vi "COD质控流程 (子VI).vi"(10 "CODMn量程切换":enum32{"H", "L", "AUTO"}(ring)=enum."AUTO", 11 "COD":bool) -> (2 "CODMn中断报警":bool, 3 "布尔":bool)   [LabVIEW 2016, in "质控单元.lvlib"]
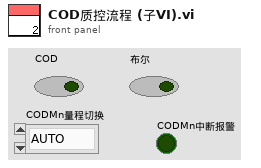
[diagram p1: front panel]
types:
  T1 = enum16{"待机", "启动水样测量", "水样测量中", "启动加标", "启动加标回收", "加标回收测量中", "结束"}
  T2 = cluster{"测量模式":enum16{"水样测量", "标样核查", "零点核查", "跨度核查", "空白测试", "加标回收", "平行样", "校零", "校标"}}
  T3 = cluster{"量程":dbl, "检出限":dbl, "加标前水样浓度":dbl, "加标后水样浓度":dbl, "加标水杯定容体积":dbl, "加标母液浓度":dbl, "加标体积":dbl, "加标回收率":dbl}
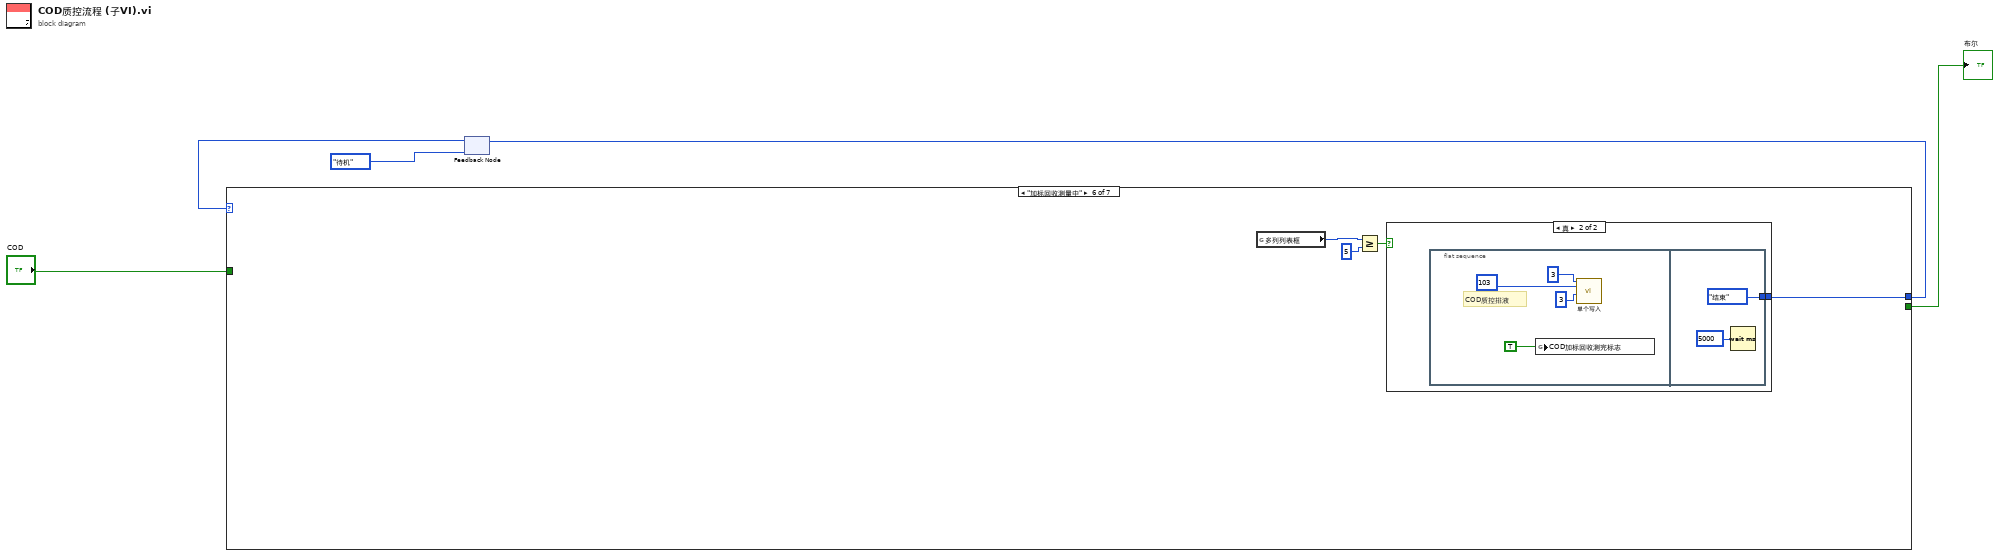
[diagram p0: block diagram]
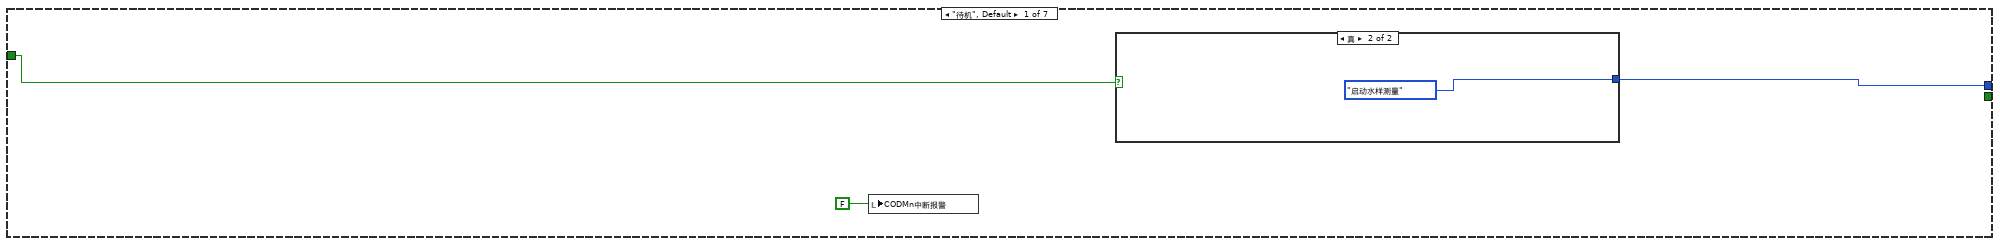
[diagram p2: hidden frame]
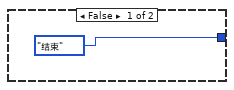
[diagram p3: hidden frame]
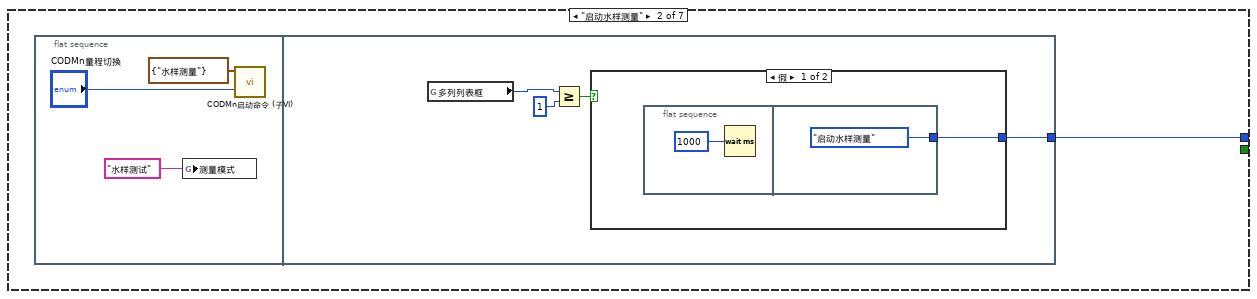
[diagram p4: hidden frame]
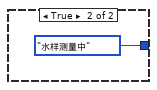
[diagram p5: hidden frame]
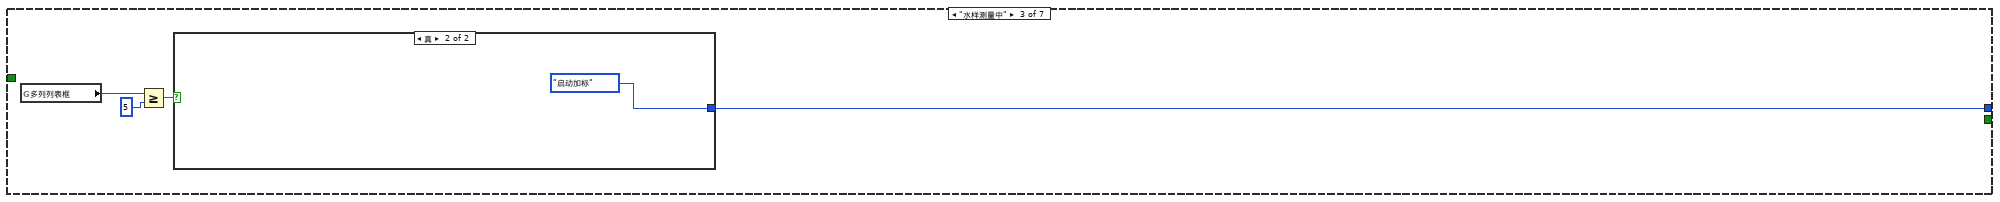
[diagram p6: hidden frame]
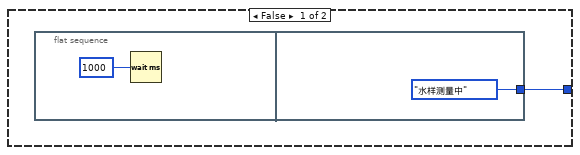
[diagram p7: hidden frame]
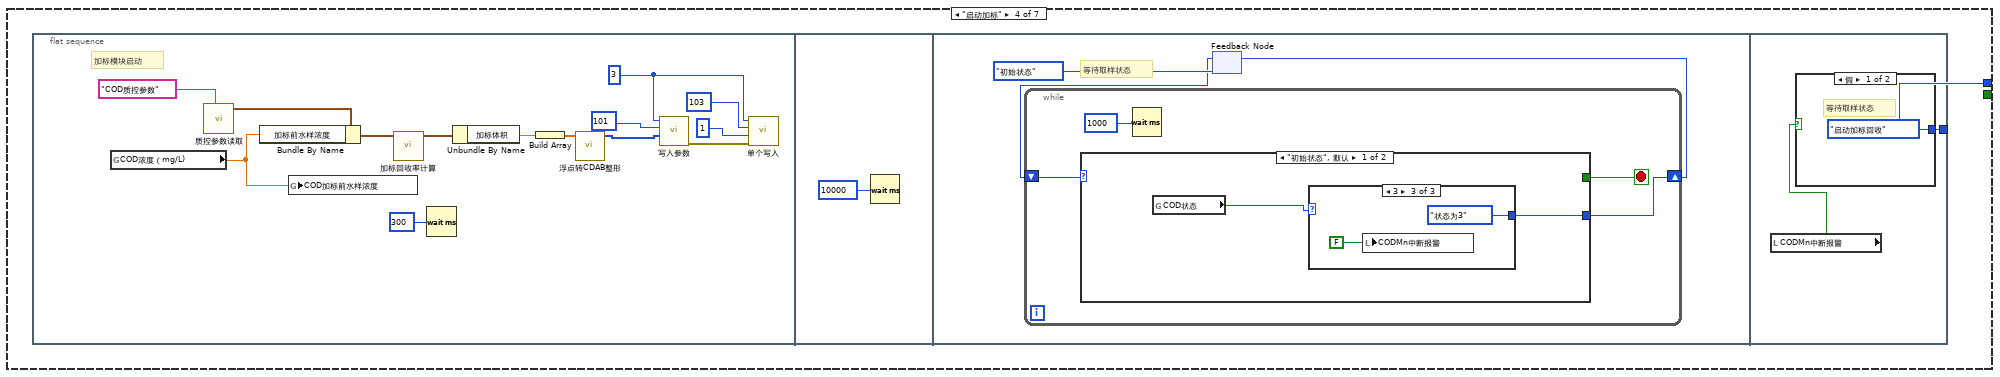
[diagram p8: hidden frame]
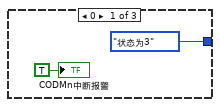
[diagram p9: hidden frame]
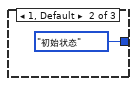
[diagram p10: hidden frame]
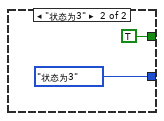
[diagram p11: hidden frame]
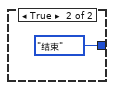
[diagram p12: hidden frame]
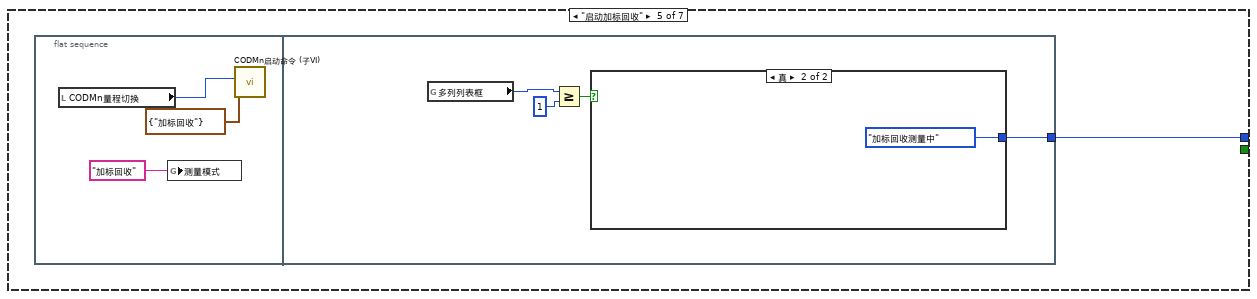
[diagram p13: hidden frame]
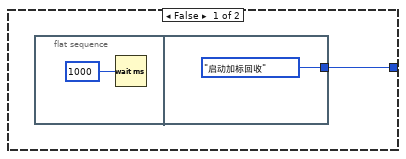
[diagram p14: hidden frame]
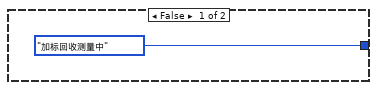
[diagram p15: hidden frame]
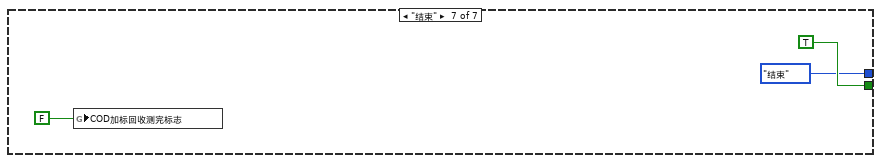
[diagram p16: hidden frame]
diagram:
  n1 = feedback #1(T1."待机") -> (w3:T1)
  n2 = case shown="\"加标回收测量中\"" w3 {
    tunnel: [w8 w11 w23 w31 w67 w79 T1."结束"] -> w4
    tunnel: [_ _ _ _ _ _ TRUE] -> w2
    tunnel: "COD" -> [w7 _ _ _ _ _ _]
    frame "待机", Default {
      n3 = local write "CODMn中断报警"(FALSE ("CODMn中断报警")) -> ()
      n4 = case shown="真" w7 {
        tunnel: [T1."结束" T1."启动水样测量"] -> w8
        frame False {
        }
        frame True {
        }
      }
    }
    frame "启动水样测量" {
      n5 = flat-sequence {
        tunnel: [w15] -> w11
        frame #0 {
          n6 = global write "COD测量模式全局.vi" "测量模式"("水样测试" ("测量模式")) -> ()
          n7 = call "CODMn启动命令 (子VI).vi"("CODMn量程切换"="CODMn量程切换", "启动测量模式"=T2 {"测量模式"=enum."水样测量"}) -> ()  [unwired: 10 in]
        }
        frame #1 {
          n8 = global read "运行时序全局变量.vi" "多列列表框"() -> (w18:i32)
          n9 = Greater Or Equal?(x=w18, y=1) -> (x >= y?=w17:bool)
          n10 = case shown="假" w17 {
            tunnel: [w19 T1."水样测量中"] -> w15
            frame False {
              n11 = flat-sequence {
                tunnel: [T1."启动水样测量"] -> w19
                frame #0 {
                  n12 = Wait (ms)(milliseconds to wait=u32 1000 ("等待时间（毫秒）")) -> ()  [unwired: 1 out]
                }
                frame #1 {
                }
              }
            }
            frame True {
            }
          }
        }
      }
    }
    frame "水样测量中" {
      n13 = global read "运行时序全局变量.vi" "多列列表框"() -> (w24:i32)
      n14 = Greater Or Equal?(x=w24, y=5) -> (x >= y?=w25:bool)
      n15 = case shown="真" w25 {
        tunnel: [w27 T1."启动加标"] -> w23
        frame False {
          n16 = flat-sequence {
            tunnel: [T1."水样测量中"] -> w27
            frame #0 {
              n17 = Wait (ms)(milliseconds to wait=u32 1000 ("等待时间（毫秒）")) -> ()  [unwired: 1 out]
            }
            frame #1 {
            }
          }
        }
        frame True {
        }
      }
    }
    frame "启动加标" {
      n18 = flat-sequence {
        tunnel: [w64] -> w31
        frame #0 {
          w33 = u16 3 ("value")
          # "加标模块启动"
          n19 = global read "COD浓度全局变量.vi" "COD浓度（mg/L)"() -> (w34:dbl)
          n20 = call "质控参数读取.vi"("section"="COD质控参数") -> ("参数"=w43:T3)  [unwired: 9 in, 1 out]
          n21 = Bundle By Name(cluster=w43, "加标前水样浓度"=w34) -> (w44:T3)
          n22 = global write "水样浓度全局.vi" "COD加标前水样浓度"(w34) -> ()
          n23 = call "加标回收率计算.vi"("参数"=w44) -> ("参数 out"=w42:T3)  [unwired: 10 in]
          n24 = Wait (ms)(milliseconds to wait=u32 300 ("等待时间（毫秒）")) -> ()  [unwired: 1 out]
          n25 = Unbundle By Name(w42) -> ("加标体积"=w35:dbl)
          n26 = Build Array(w35) -> (w41:dbl[])
          n27 = call "浮点转CDAB整形.vi"("浮点数"=w41) -> ("CDAB整形输出"=w36:u16[])  [unwired: 10 in]
          n28 = call "写入参数.vi"("values"=w36, "starting address"=u16 101, "Slave ID"=w33) -> ("error out"=w40:errorcluster)  [unwired: 8 in]
          n29 = call "单个写入.vi"("Error in"=w40, "value"=u16 1, "address"=u16 103, "Slave ID"=w33) -> ()  [unwired: 7 in, 1 out]
        }
        frame #1 {
          n30 = Wait (ms)(milliseconds to wait=u32 10000 ("等待时间（毫秒）")) -> ()  [unwired: 1 out]
        }
        frame #2 {
          # "等待取样状态"
          n31 = feedback #2(enum16{"初始状态", "状态为3"}."初始状态") -> (w48:enum16{"初始状态", "状态为3"})
          n32 = while {
            shift-right: [w52] -> w47
            shift-left: w48 -> [w53]
            stop <- w51 stop-if-true
            n33 = case shown="\"初始状态\", 默认" w53 {
              tunnel: [w55 enum16{"初始状态", "状态为3"}."状态为3"] -> w52
              tunnel: [_ TRUE] -> w51
              frame "初始状态", Default {
                n34 = global read "氨氮加标回收状态全局变量.vi" "COD状态"() -> (w54:u16)
                n35 = case shown="3" w54 {
                  tunnel: [enum16{"初始状态", "状态为3"}."状态为3" enum16{"初始状态", "状态为3"}."初始状态" enum16{"初始状态", "状态为3"}."状态为3"] -> w55
                  frame 0 {
                    "CODMn中断报警" <- TRUE ("CODMn中断报警")
                  }
                  frame 1, Default {
                  }
                  frame 3 {
                    n36 = local write "CODMn中断报警"(FALSE ("CODMn中断报警")) -> ()
                  }
                }
              }
              frame "状态为3" {
              }
            }
            n37 = Wait (ms)(milliseconds to wait=u32 1000 ("等待时间（毫秒）")) -> ()  [unwired: 1 out]
          }
          n38 = feedback-in #2(w47) -> ()
        }
        frame #3 {
          n39 = local read "CODMn中断报警"() -> (w63:bool)
          n40 = case shown="假" w63 {
            tunnel: [T1."启动加标回收" T1."结束"] -> w64
            frame False {
              # "等待取样状态"
            }
            frame True {
            }
          }
        }
      }
    }
    frame "启动加标回收" {
      n41 = flat-sequence {
        tunnel: [w71] -> w67
        frame #0 {
          n42 = local read "CODMn量程切换"() -> (w69:enum32{"H", "L", "AUTO"})
          n43 = global write "COD测量模式全局.vi" "测量模式"("加标回收" ("测量模式")) -> ()
          n44 = call "CODMn启动命令 (子VI).vi"("CODMn量程切换"=w69, "启动测量模式"=T2 {"测量模式"=enum."加标回收"}) -> ()  [unwired: 10 in]
        }
        frame #1 {
          n45 = global read "运行时序全局变量.vi" "多列列表框"() -> (w72:i32)
          n46 = Greater Or Equal?(x=w72, y=1) -> (x >= y?=w73:bool)
          n47 = case shown="真" w73 {
            tunnel: [w75 T1."加标回收测量中"] -> w71
            frame False {
              n48 = flat-sequence {
                tunnel: [T1."启动加标回收"] -> w75
                frame #0 {
                  n49 = Wait (ms)(milliseconds to wait=u32 1000 ("等待时间（毫秒）")) -> ()  [unwired: 1 out]
                }
                frame #1 {
                }
              }
            }
            frame True {
            }
          }
        }
      }
    }
    frame "加标回收测量中" {
      n50 = global read "运行时序全局变量.vi" "多列列表框"() -> (w80:i32)
      n51 = Greater Or Equal?(x=w80, y=5) -> (x >= y?=w81:bool)
      n52 = case shown="真" w81 {
        tunnel: [T1."加标回收测量中" w84] -> w79
        frame False {
        }
        frame True {
          n53 = flat-sequence {
            tunnel: [T1."结束"] -> w84
            frame #0 {
              # "COD质控排液"
              n54 = global write "质控测完标志全局 1.vi" "COD加标回收测完标志"(TRUE ("COD加标回收测完标志")) -> ()
              n55 = call "单个写入.vi"("value"=u16 3, "address"=u16 103, "Slave ID"=u8 3) -> ()  [unwired: 8 in, 1 out]
            }
            frame #1 {
              n56 = Wait (ms)(milliseconds to wait=u32 5000 ("等待时间（毫秒）")) -> ()  [unwired: 1 out]
            }
          }
        }
      }
    }
    frame "结束" {
      n57 = global write "质控测完标志全局 1.vi" "COD加标回收测完标志"(FALSE ("COD加标回收测完标志")) -> ()
    }
  }
  "布尔" <- w2
  n58 = feedback-in #1(w4) -> ()
